vi "DrawTable.vi"(0 "Table":refnum<vi>, 1 "cfg":T1, 2 "Array":cluster{bool[], string[]}[](array[cluster])) -> ()   [LabVIEW 2018]
uses:
  ControlCfg.ctl
  ControlConfigMisura.ctl
  ControlConfigDI.ctl
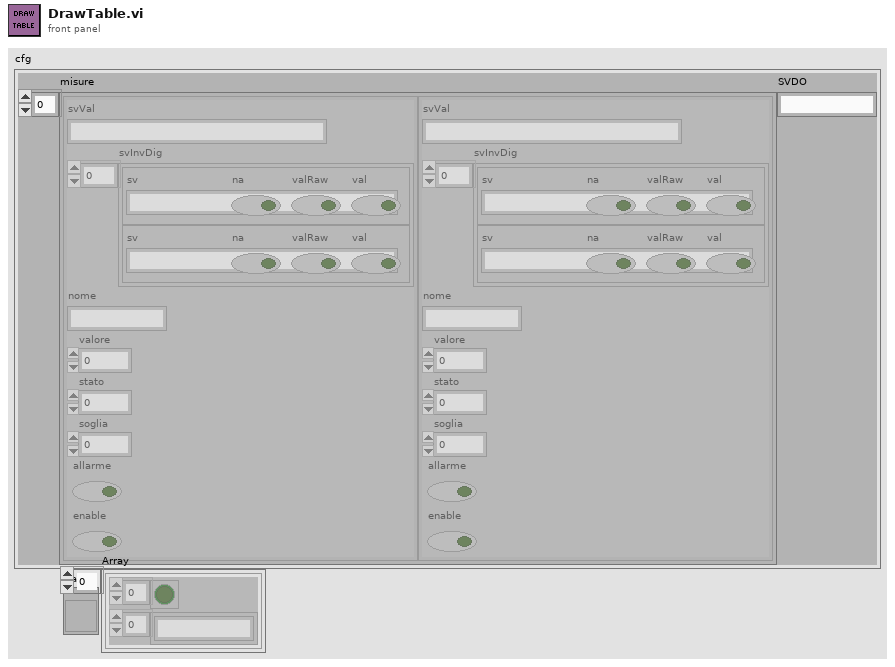
[diagram p1: front panel]
types:
  T1 = typedef "ControlCfg.ctl" = cluster{"misure":T2[], "SVDO":string}
  T2 = typedef "ControlConfigMisura.ctl" = cluster{"svVal":string, "svInvDig":T3[], "nome":string, "valore":dbl, "stato":i16, "soglia":dbl, "allarme":bool, "enable":bool}
  T3 = typedef "ControlConfigDI.ctl" = cluster{"sv":string, "na":bool, "valRaw":bool, "val":bool}
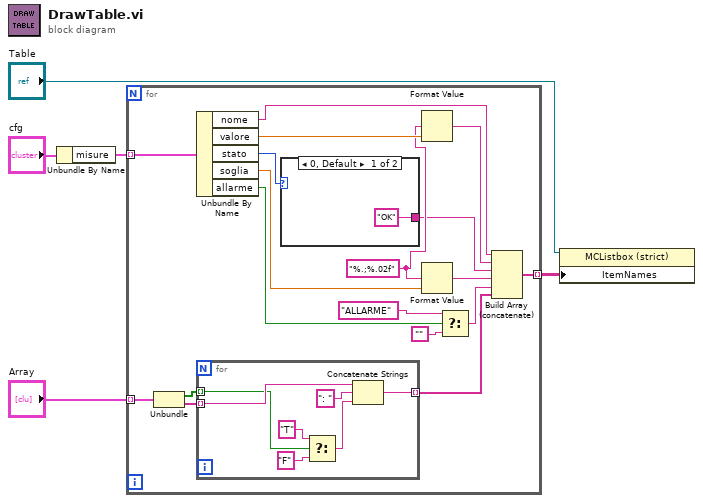
[diagram p0: block diagram]
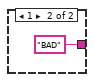
[diagram p2: hidden frame]
diagram:
  n1 = Unbundle By Name("cfg") -> ("misure"=w4:T2[])
  n2 = for {
    tunnel: w4 -> [w23] mode=indexing
    tunnel: [w10] -> w3 mode=indexing
    tunnel: "Array" -> [w9] mode=indexing
    w20 = "%.;%.02f" ("format string")
    n3 = Unbundle(w9) -> (w7:bool[], w8:string[])
    n4 = Unbundle By Name(w23) -> ("nome"=w19:string, "valore"=w22:dbl, "stato"=w14:i16, "soglia"=w21:dbl, "allarme"=w17:bool)
    n5 = for {
      tunnel: w8 -> [w30] mode=indexing
      tunnel: w7 -> [w28] mode=indexing
      tunnel: [w24] -> w6 mode=indexing
      n6 = Select(t="T" ("string"), s=w28, f="F" ("string")) -> (s? t:f=w25:string)
      n7 = Concatenate Strings(w30, ": " ("string"), w25) -> (w24:string)
    }
    n8 = case shown="0, Default" w14 {
      tunnel: ["OK" "BAD"] -> w13
      frame 0, Default {
      }
      frame 1 {
      }
    }
    n9 = Format Value(format string=w20, value (0)=w22) -> (output string=w18:string)  [unwired: 1 in]
    n10 = Format Value(format string=w20, value (0)=w21) -> (output string=w12:string)  [unwired: 1 in]
    n11 = Select(t="ALLARME", s=w17, f="") -> (s? t:f=w11:string)
    n12 = Build Array (concatenate)(w19, w18, w13, w12, w11, w6) -> (w10:string[])
  }
  n13 = property class="MCListbox (strict)"(reference="Table", "ItemNames"=w3) -> ()  [unwired: 1 in, 2 out]
